vi "Execute Services.vi"(8 "error in (no error)":errorcluster, 11 "Manejo Turnos in":refnum<class "Manejo Turnos.lvclass">) -> (0 "error out":errorcluster, 3 "Manejo Turnos out":refnum<class "Manejo Turnos.lvclass">)   [LabVIEW 2020, in "Manejo Turnos.lvlib" / "Manejo Turnos.lvclass"]
uses:
  Manejo Turnos.lvclass
  C:/Program Files (x86)/National Instruments/LabVIEW 2020/vi.lib/ActorFramework/Actor/Actor.lvclass
  Manejo Turnos.lvclass/Manejo Turnos.ctl
  <vilib>/ActorFramework/Actor/Actor.lvclass/Actor.ctl
  <vilib>/ActorFramework/Message Enqueuer/Message Enqueuer.lvclass/Message Enqueuer.ctl
  <vilib>/ActorFramework/Message Enqueuer/Init from Existing Queue.vi
  <vilib>/ActorFramework/Message Enqueuer/Enqueue.vi
  Manejo Turnos Messages/Wax Service Msg/Wax Service Msg.lvclass
  C:/Program Files (x86)/National Instruments/LabVIEW 2020/vi.lib/ActorFramework/Message/Message.lvclass
  Manejo Turnos Messages/Taxi Service Msg/Taxi Service Msg.lvclass
  Manejo Turnos Messages/Motor Service Msg/Motor Service Msg.lvclass
  Manejo Turnos Messages/Basic Service Msg/Basic Service Msg.lvclass
  Manejo Turnos Messages/Total Service Msg/Total Service Msg.lvclass
  <vilib>/ActorFramework/Message Priority Queue/Priority Enqueue.vi
  <vilib>/ActorFramework/Message Enqueuer/Message Enqueuer.lvclass
  <vilib>/ActorFramework/Actor/Actor.lvclass
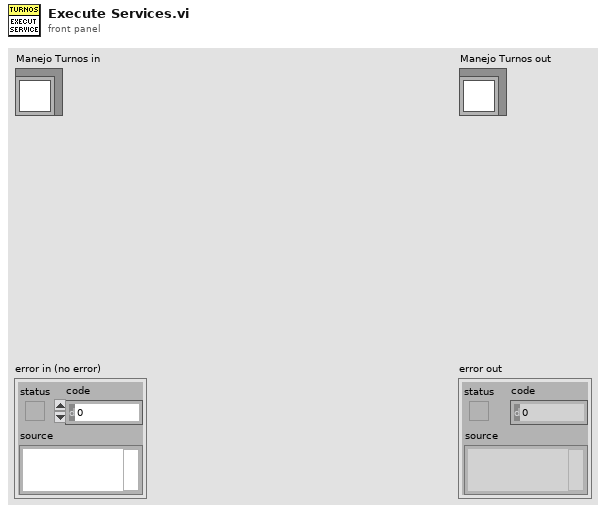
[diagram p1: front panel]
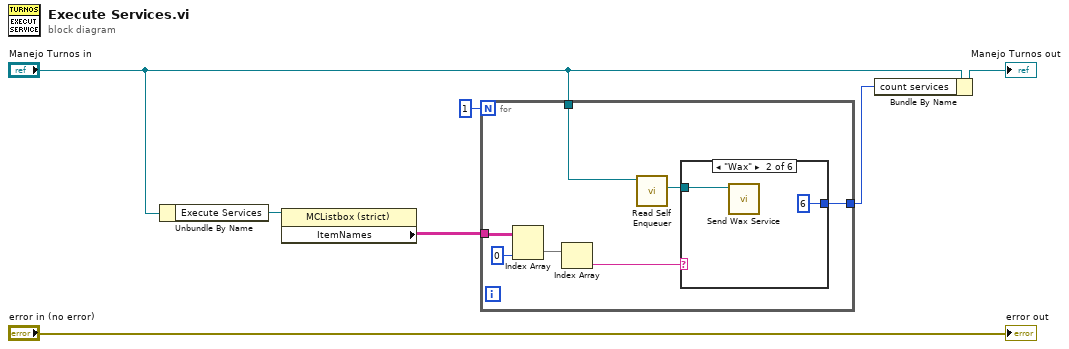
[diagram p0: block diagram]
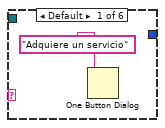
[diagram p2: hidden frame]
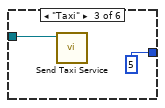
[diagram p3: hidden frame]
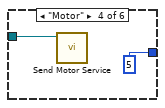
[diagram p4: hidden frame]
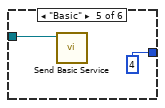
[diagram p5: hidden frame]
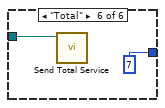
[diagram p6: hidden frame]
diagram:
  n1 = Unbundle By Name("Manejo Turnos in") -> ("Execute Services"=w6:refnum<vi>)
  n2 = property class="MCListbox (strict)"(reference=w6) -> ("ItemNames"=w3:string[][])  [unwired: 1 in, 2 out]
  n3 = for {
    N: 1 -> [_]
    tunnel: "Manejo Turnos in" -> [w8]
    tunnel: w3 -> [w10]
    tunnel: [w9] -> w1
    n4 = Index Array(array=w10, index (col)=0 ("index (row)")) -> (element=w13:string[])  [unwired: 1 in]
    n5 = Index Array(array=w13) -> (element=w12:string)  [unwired: 1 in]
    n6 = call <vilib>:"Read Self Enqueuer.vi"("Actor"=w8) -> ("Self Enqueuer"=w11:refnum<class "Message Enqueuer.lvclass">)  [unwired: 10 in]
    n7 = case shown="\"Wax\"" w12 {
      tunnel: w11 -> [_ w17 w19 w21 w23 w25]
      tunnel: [_ 6 5 5 4 7] -> w9
      frame Default {
        n8 = One Button Dialog(message="Adquiere un servicio") -> ()  [unwired: 1 in, 1 out]
      }
      frame "Wax" {
        n9 = call "Send Wax Service.vi"("Message Enqueuer"=w17) -> ()  [unwired: 9 in, 2 out]
      }
      frame "Taxi" {
        n10 = call "Send Taxi Service.vi"("Message Enqueuer"=w19) -> ()  [unwired: 9 in, 2 out]
      }
      frame "Motor" {
        n11 = call "Send Motor Service.vi"("Message Enqueuer"=w21) -> ()  [unwired: 9 in, 2 out]
      }
      frame "Basic" {
        n12 = call "Send Basic Service.vi"("Message Enqueuer"=w23) -> ()  [unwired: 9 in, 2 out]
      }
      frame "Total" {
        n13 = call "Send Total Service.vi"("Message Enqueuer"=w25) -> ()  [unwired: 9 in, 2 out]
      }
    }
  }
  n14 = Bundle By Name(cluster="Manejo Turnos in", "count services"=w1) -> (→"Manejo Turnos out":refnum<class "Manejo Turnos.lvclass">)
  "error out" <- "error in (no error)"
